vi "setTwoToneSignal.vi"(7 "Channel":string="0", 8 "error in (no error)":errorcluster, 9 "tone amplitudes":dbl format="%.2p", 10 "tone frequencies":dbl format="%.2p", 11 "FgenKeysight in":refnum<class "ArbKeysight.lvclass">) -> (0 "error out":errorcluster, 3 "FgenKeysight out":refnum<class "ArbKeysight.lvclass">)   [LabVIEW 2023, in "ArbKeysight.lvclass"]
doc: "<b>Author:</b> Wolfgang\n<b>Description:</b> Apply a two tone signal"
uses:
  ArbKeysight.lvclass
  Arb.lvclass
  Data/arbWaveformType.ctl
  Driver/Keysight-33500B.lvlib
  sweArb.lvlib
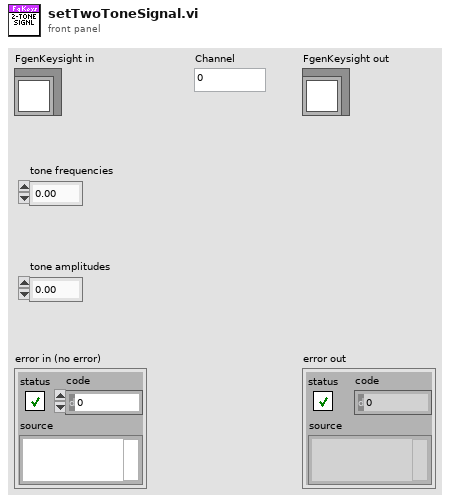
[diagram p1: front panel]
types:
  T1 = typedef "sweArb.lvlib/arbWaveformType.ctl" = enum16{"Sine", "Square", "Triangle", "DC", "Noise", "Arb"}
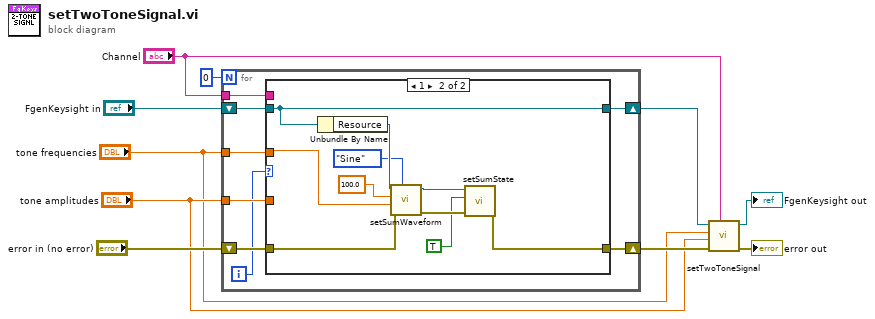
[diagram p0: block diagram]
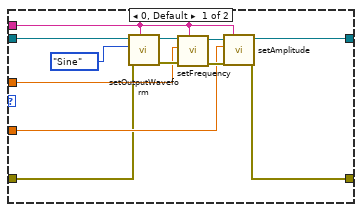
[diagram p2: hidden frame]
diagram:
  n1 = for {
    N: 0 -> [_]
    tunnel: "Channel" -> [w16]
    shift-right: [w17] -> w7
    shift-left: "FgenKeysight in" -> [w18]
    tunnel: "tone frequencies" -> [w14]
    tunnel: "tone amplitudes" -> [w15]
    shift-right: [w12] -> w4
    shift-left: "error in (no error)" -> [w13]
    i -> [w11]
    n2 = case shown="1" w11 {
      tunnel: w18 -> [w30 w32]
      tunnel: [w27 w32] -> w17
      tunnel: w16 -> [w24 _]
      tunnel: w15 -> [w23 _]
      tunnel: w14 -> [w22 w38]
      tunnel: w13 -> [w20 w37]
      tunnel: [w19 w34] -> w12
      frame 0, Default {
        n3 = call-dynamic "setOutputWaveform.vi"("Channel"=w24, "error in (no error)"=w20, "Type"=arbWaveformType."Sine", "FgenKeysight in"=w30) -> ("error out"=w26:errorcluster, "FgenKeysight out"=w29:refnum<class "ArbKeysight.lvclass">)  [unwired: 6 in]
        n4 = call-dynamic "setFrequency.vi"("Channel"=w24, "error in (no error)"=w26, "Frequency [Hz]"=w22, "FgenKeysight in"=w29) -> ("error out"=w25:errorcluster, "FgenKeysight out"=w28:refnum<class "ArbKeysight.lvclass">)  [unwired: 6 in]
        n5 = call-dynamic "setAmplitude.vi"("Channel"=w24, "error in (no error)"=w25, "Amplitude [Vpkpk]"=w23, "FgenKeysight in"=w28) -> ("error out"=w19:errorcluster, "FgenKeysight out"=w27:refnum<class "ArbKeysight.lvclass">)  [unwired: 6 in]
      }
      frame 1 {
        n6 = Unbundle By Name(w32) -> ("Resource"=w40:refnum<visa-resource-name>)
        n7 = call "setSumWaveform.vi"("Waveform"=enum16{"Sine", "Rectangular", "Triangular"}."Sine", "error in (no error)"=w37, "Frequency [Hz]"=w38, "Amplitude [%]"=100.0, "VISA resource name"=w40) -> ("error out"=w36:errorcluster, "VISA resource name out"=w35:refnum<visa-resource-name>)  [unwired: 5 in]
        n8 = call "setSumState.vi"("error in (no error)"=w36, "State"=TRUE, "VISA resource name"=w35) -> ("error out"=w34:errorcluster)  [unwired: 7 in, 1 out]
      }
    }
  }
  n9 = call-parent "setTwoToneSignal.vi"("Channel"="Channel", "error in (no error)"=w4, "tone amplitudes"="tone amplitudes", "tone frequencies"="tone frequencies", "Fgen.lvclass"=w7) -> ("error out"=→"error out":errorcluster, "Fgen.lvclass out"=→"FgenKeysight out":refnum<class "ArbKeysight.lvclass">)  [unwired: 5 in]
